vi "Constant.vi"() -> ()   [LabVIEW 2019]
panel:
  out "Circumference":dbl
  in  "Radius":dbl
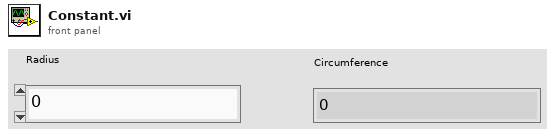
[diagram p1: front panel]
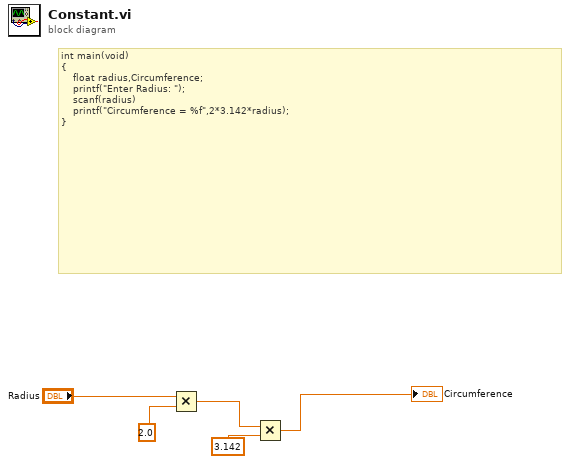
[diagram p0: block diagram]
diagram:
  # "int main(void)\n{\n    float radius,Circumference;\n    printf(\"Enter Radius: \");\n    scanf(radius) \n    printf(\"Circumference = %f\",2*3.142*radius);\n}"
  n1 = Multiply(x="Radius", y=2.0) -> (x*y=w3:dbl)
  n2 = Multiply(x=w3, y=3.142) -> (x*y=→"Circumference":dbl)
